vi "写入-剂量率.vi"(8 "error in (no error)":errorcluster caption="错误输入（无错误）", 10 "剂量率":cluster{"剂量率":dbl, "时间":timestamp}, 11 "设备终端输入":refnum<class "设备终端.lvclass">) -> (0 "error out":errorcluster caption="错误输出", 3 "设备终端输出":refnum<class "设备终端.lvclass">)   [LabVIEW 2013, in "设备终端.lvclass"]
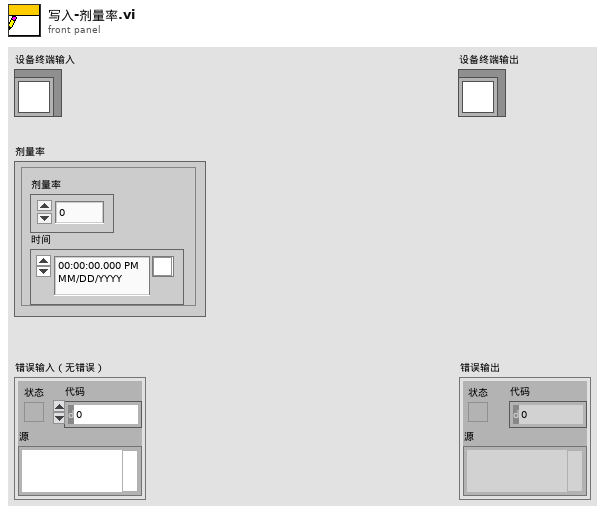
[diagram p1: front panel]
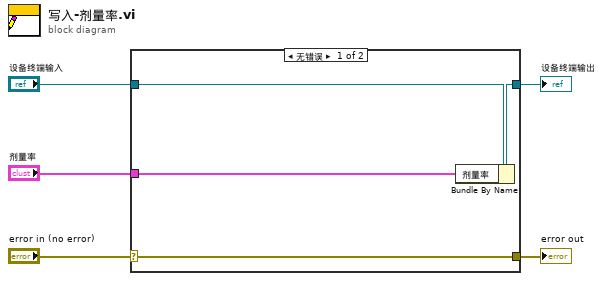
[diagram p0: block diagram]
diagram:
  n1 = case shown="无错误" "error in (no error)" {
    selector: "error in (no error)" -> [w9 w10]
    tunnel: [w9 w10] -> w4
    tunnel: [w7 w11] -> w2
    tunnel: "设备终端输入" -> [w8 w11]
    tunnel: "剂量率" -> [w6 _]
    frame No Error {
      n2 = Bundle By Name(cluster=w8, "剂量率"=w6) -> (w7:refnum<class "设备终端.lvclass">)
    }
    frame Error {
    }
  }
  "error out" <- w4
  "设备终端输出" <- w2
